vi "NISE.remote.Reset Devices.vi"(0 "SLSC Remote in":refnum<class "SLSC Interface.lvclass">, 5 "devices":refnum<k21>="$DefaultDevices", 11 "error in (no error)":errorcluster) -> (4 "SLSC Remote out":refnum<class "SLSC Interface.lvclass">, 15 "error out":errorcluster)   [LabVIEW 2016, in "SLSC Interface.lvclass"]
uses:
  SLSC Interface Class/SLSC Interface.lvclass
  SLSC Interface Class/SLSC Interface.lvclass/SLSC Interface.ctl
  SLSC Interface Class/NISE.Read client handle.vi
  SLSC Interface Class/NISE.Read URL.vi
  SLSC Interface Class/NISE.Read session.vi
  <vilib>/httpClient/POSTBuffer.vi
  <vilib>/httpClient/LabVIEWHTTPClient.lvlib
  <vilib>/NI/JSON Support for LabVIEW/JSON Value/JSON Value.lvclass
  <vilib>/NI/NI JSONRPC Server Framework/Classes/Client/JSONRPC Client.lvclass
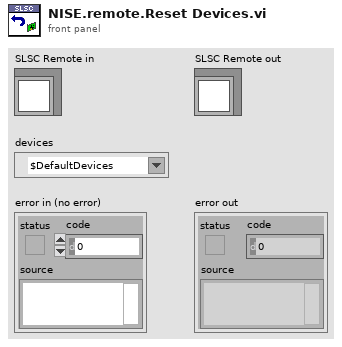
[diagram p1: front panel]
types:
  T1 = typedef "LabVIEWHTTPClient.lvlib/ClientHandle.ctl" = refnum<k1>
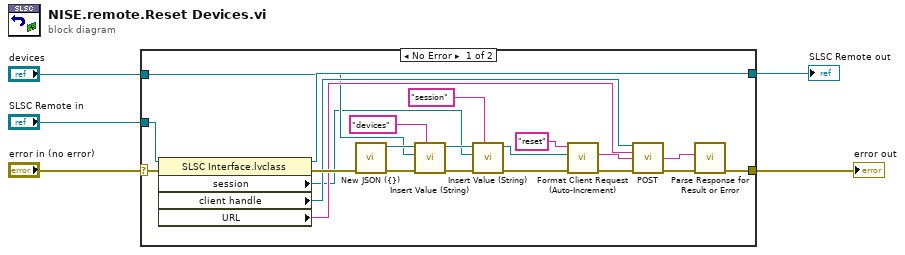
[diagram p0: block diagram]
diagram:
  n1 = case shown="No Error" "error in (no error)" {
    selector: "error in (no error)" -> [w25 w28]
    tunnel: "devices" -> [w7 _]
    tunnel: "SLSC Remote in" -> [w27 w29]
    tunnel: [w26 w29] -> w3
    tunnel: [w12 w28] -> w2
    frame No Error {
      n2 = property class="SLSC Interface.lvclass"(reference=w27, error in=w25) -> (reference out=w26:refnum<class "SLSC Interface.lvclass">, error out=w24:errorcluster, "session"=w6:refnum<k21>, "client handle"=w17:T1, "URL"=w16:string)
      n3 = call <vilib>:"New JSON ({}).vi"("error in (no error)"=w24) -> ("error out"=w23:errorcluster, "JSON Value out"=w11:refnum<class "JSON Value.lvclass">)  [unwired: 9 in]
      n4 = call <vilib>:"Insert Value (String).vi"("key"="devices" ("Name"), "error in (no error)"=w23, "value"=w7, "JSON Value in"=w11) -> ("error out"=w22:errorcluster, "JSON Value out"=w10:refnum<class "JSON Value.lvclass">)  [unwired: 5 in, 1 out]
      n5 = call <vilib>:"Insert Value (String).vi"("key"="session" ("Name"), "error in (no error)"=w22, "value"=w6, "JSON Value in"=w10) -> ("error out"=w18:errorcluster, "JSON Value out"=w19:refnum<class "JSON Value.lvclass">)  [unwired: 5 in, 1 out]
      n6 = call <vilib>:"Format Client Request (Auto-Increment).vi"("error in (no error)"=w18, "JSON Value in"=w19, "method"="reset") -> ("error out"=w15:errorcluster, "Request String"=w20:string)  [unwired: 7 in]
      n7 = call-poly <vilib>:"POST.vi"("client handle"=w17, "url"=w16, "buffer"=w20, "error in (no error)"=w15) -> ("body"=w14:string, "error out"=w13:errorcluster)  [unwired: 8 in, 2 out]
      n8 = call <vilib>:"Parse Response for Result or Error.vi"("error in"=w13, "Response String In"=w14) -> ("error out"=w12:errorcluster)  [unwired: 7 in, 2 out]
    }
    frame Error {
    }
  }
  "error out" <- w2
  "SLSC Remote out" <- w3
